vi "Shuffle 360.vi"(8 "error in (no error)":errorcluster, 11 "Board in":refnum<class "Board.lvclass">) -> (0 "error out":errorcluster, 3 "Board out":refnum<class "Board.lvclass">)   [LabVIEW 2021, in "Board.lvclass"]
uses:
  Board.lvclass
  Board.lvclass/Board.ctl
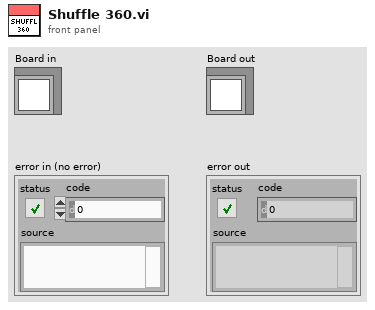
[diagram p1: front panel]
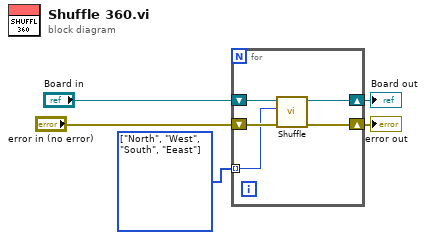
[diagram p0: block diagram]
diagram:
  w5 = enum16{"North", "Eeast", "South", "West"}[] [enum."North", enum."West", enum."South", enum."Eeast"] items=["North", "Eeast", "South", "West"] ("North")
  n1 = for {
    shift-right: [w8] -> w3
    shift-left: "error in (no error)" -> [w10]
    shift-right: [w7] -> w4
    shift-left: "Board in" -> [w9]
    tunnel: w5 -> [w6] mode=indexing
    n2 = call "Shuffle.vi"("error in (no error)"=w10, "North"=w6, "Proto in"=w9) -> ("error out"=w8:errorcluster, "Proto out"=w7:refnum<class "Board.lvclass">)  [unwired: 7 in]
  }
  "Board out" <- w4
  "error out" <- w3
